vi "Decode BMS Packet.vi"(10 "Array":u8[](array[numeric])) -> (2 "xml string":string)   [LabVIEW 2014]
uses:
  BMS Telemetry.ctl
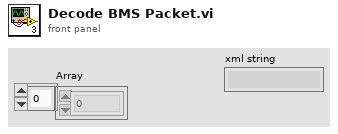
[diagram p1: front panel]
types:
  T1 = typedef "BMS Telemetry.ctl" = cluster{"bBMSIgnition":bool, "bBMSChargerMains":bool, "bBMSFastCharge":bool, "bBMSChargerEnabled":bool, "eBMSCarState":enum16{"Off", "On, Not Charging", "Charging", "Charging Finished", "Charging Error"}, "eBMSChargingState":enum16{"Disconnected", "Pre-charging", "Main Charging", "Balancing", "Charging Finished OK", "Charging Error"}, "tBMSChargeStage":u16, "eBMSLastChargeError":enum16{"No Error", "Cell Voltage Too Low", "No Comm from Cells so can't start", "Maximum charging stage duration expired", "No Comm from Cels so can't balande", "Cannot set balancing voltage", "Cell temps too high", "No Comms so can't determine temp", "# of Cells Mismatch", "Cells Overvoltage", "Cell Protection Event occured."}, "NBMSNumCells":u8, "bBMSUnderVProtection":bool, "bBMSOverVProtection":bool, "bBMSOverTProtection":bool, "bBMSLeakageProtection":bool, "bBMSNoCellCommsError":bool, "bBMSLowVReduction":bool, "bBMSHighTReduction":bool, "VCellMin":dbl, "VCellMax":dbl, "VCellMean":dbl, "VTotal":dbl, "TCellMin":dbl, "TCellMax":dbl, "TCellMean":dbl, "VCells":cluster{"[51]":dbl, "[52]":dbl, "[53]":dbl, "[54]":dbl, "[55]":dbl, "[56]":dbl, "[57]":dbl, "[58]":dbl, "[59]":dbl, "[60]":dbl, "[61]":dbl, "[62]":dbl, "[63]":dbl, "[64]":dbl, "[65]":dbl, "[66]":dbl, "[67]":dbl, "[34]":dbl, "[35]":dbl, "[36]":dbl, "[37]":dbl, "[38]":dbl, "[39]":dbl, "[40]":dbl, "[41]":dbl, "[42]":dbl, "[43]":dbl, "[44]":dbl, "[45]":dbl, "[46]":dbl, "[47]":dbl, "[48]":dbl, "[49]":dbl, "[50]":dbl, "[17]":dbl, "[18]":dbl, "[19]":dbl, "[20]":dbl, "[21]":dbl, "[22]":dbl, "[23]":dbl, "[24]":dbl, "[25]":dbl, "[26]":dbl, "[27]":dbl, "[28]":dbl, "[29]":dbl, "[30]":dbl, "[31]":dbl, "[32]":dbl, "[33]":dbl, "[0]":dbl, "[1]":dbl, "[2]":dbl, "[3]":dbl, "[4]":dbl, "[5]":dbl, "[6]":dbl, "[7]":dbl, "[8]":dbl, "[9]":dbl, "[10]":dbl, "[11]":dbl, "[12]":dbl, "[13]":dbl, "[14]":dbl, "[15]":dbl, "[16]":dbl}, "TCells":cluster{"[55]":dbl, "[56]":dbl, "[57]":dbl, "[58]":dbl, "[59]":dbl, "[60]":dbl, "[61]":dbl, "[62]":dbl, "[63]":dbl, "[64]":dbl, "[65]":dbl, "[66]":dbl, "[67]":dbl, "[68]":dbl, "[69]":dbl, "[70]":dbl, "[17]":dbl, "[38]":dbl, "[39]":dbl, "[40]":dbl, "[41]":dbl, "[42]":dbl, "[43]":dbl, "[44]":dbl, "[45]":dbl, "[46]":dbl, "[47]":dbl, "[48]":dbl, "[49]":dbl, "[50]":dbl, "[51]":dbl, "[52]":dbl, "[53]":dbl, "[54]":dbl, "[21]":dbl, "[22]":dbl, "[23]":dbl, "[24]":dbl, "[25]":dbl, "[26]":dbl, "[27]":dbl, "[28]":dbl, "[29]":dbl, "[30]":dbl, "[31]":dbl, "[32]":dbl, "[33]":dbl, "[34]":dbl, "[35]":dbl, "[36]":dbl, "[37]":dbl, "[0]":dbl, "[1]":dbl, "[2]":dbl, "[3]":dbl, "[4]":dbl, "[5]":dbl, "[6]":dbl, "[7]":dbl, "[8]":dbl, "[9]":dbl, "[10]":dbl, "[11]":dbl, "[12]":dbl, "[13]":dbl, "[14]":dbl, "[15]":dbl, "[16]":dbl}}
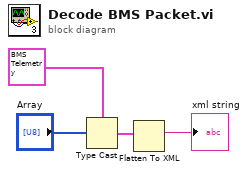
[diagram p0: block diagram]
diagram:
  n1 = Type Cast(type=T1 {"bBMSIgnition"=FALSE, "bBMSChargerMains"=FALSE, "bBMSFastCharge"=FALSE, "bBMSChargerEnabled"=FALSE, "eBMSCarState"=enum."Off", "eBMSChargingState"=enum."Disconnected", "tBMSChargeStage"=0, "eBMSLastChargeError"=enum."No Error", "NBMSNumCells"=0, "bBMSUnderVProtection"=FALSE, "bBMSOverVProtection"=FALSE, "bBMSOverTProtection"=FALSE, "bBMSLeakageProtection"=FALSE, "bBMSNoCellCommsError"=FALSE, "bBMSLowVReduction"=FALSE, "bBMSHighTReduction"=FALSE, "VCellMin"=0.0, "VCellMax"=0.0, "VCellMean"=0.0, "VTotal"=0.0, "TCellMin"=0.0, "TCellMax"=0.0, "TCellMean"=0.0, "VCells"={"[51]"=0.0, "[52]"=0.0, "[53]"=0.0, "[54]"=0.0, "[55]"=0.0, "[56]"=0.0, "[57]"=0.0, "[58]"=0.0, "[59]"=0.0, "[60]"=0.0, "[61]"=0.0, "[62]"=0.0, "[63]"=0.0, "[64]"=0.0, "[65]"=0.0, "[66]"=0.0, "[67]"=0.0, "[34]"=0.0, "[35]"=0.0, "[36]"=0.0, "[37]"=0.0, "[38]"=0.0, "[39]"=0.0, "[40]"=0.0, "[41]"=0.0, "[42]"=0.0, "[43]"=0.0, "[44]"=0.0, "[45]"=0.0, "[46]"=0.0, "[47]"=0.0, "[48]"=0.0, "[49]"=0.0, "[50]"=0.0, "[17]"=0.0, "[18]"=0.0, "[19]"=0.0, "[20]"=0.0, "[21]"=0.0, "[22]"=0.0, "[23]"=0.0, "[24]"=0.0, "[25]"=0.0, "[26]"=0.0, "[27]"=0.0, "[28]"=0.0, "[29]"=0.0, "[30]"=0.0, "[31]"=0.0, "[32]"=0.0, "[33]"=0.0, "[0]"=0.0, "[1]"=0.0, "[2]"=0.0, "[3]"=0.0, "[4]"=0.0, "[5]"=0.0, "[6]"=0.0, "[7]"=0.0, "[8]"=0.0, "[9]"=0.0, "[10]"=0.0, "[11]"=0.0, "[12]"=0.0, "[13]"=0.0, "[14]"=0.0, "[15]"=0.0, "[16]"=0.0}, "TCells"={"[55]"=0.0, "[56]"=0.0, "[57]"=0.0, "[58]"=0.0, "[59]"=0.0, "[60]"=0.0, "[61]"=0.0, "[62]"=0.0, "[63]"=0.0, "[64]"=0.0, "[65]"=0.0, "[66]"=0.0, "[67]"=0.0, "[68]"=0.0, "[69]"=0.0, "[70]"=0.0, "[17]"=0.0, "[38]"=0.0, "[39]"=0.0, "[40]"=0.0, "[41]"=0.0, "[42]"=0.0, "[43]"=0.0, "[44]"=0.0, "[45]"=0.0, "[46]"=0.0, "[47]"=0.0, "[48]"=0.0, "[49]"=0.0, "[50]"=0.0, "[51]"=0.0, "[52]"=0.0, "[53]"=0.0, "[54]"=0.0, "[21]"=0.0, "[22]"=0.0, "[23]"=0.0, "[24]"=0.0, "[25]"=0.0, "[26]"=0.0, "[27]"=0.0, "[28]"=0.0, "[29]"=0.0, "[30]"=0.0, "[31]"=0.0, "[32]"=0.0, "[33]"=0.0, "[34]"=0.0, "[35]"=0.0, "[36]"=0.0, "[37]"=0.0, "[0]"=0.0, "[1]"=0.0, "[2]"=0.0, "[3]"=0.0, "[4]"=0.0, "[5]"=0.0, "[6]"=0.0, "[7]"=0.0, "[8]"=0.0, "[9]"=0.0, "[10]"=0.0, "[11]"=0.0, "[12]"=0.0, "[13]"=0.0, "[14]"=0.0, "[15]"=0.0, "[16]"=0.0}} ("BMS Telemetry"), x="Array") -> (*(type *) &x=w3:T1)
  n2 = Flatten To XML(anything=w3) -> (xml string=→"xml string":string)
